vi "Fix File Name.vi"(11 "Config Name":string) -> (3 "File Name":string)   [LabVIEW 2020, in "Negentropic IDE.lvlib"]
uses:
  Negentropic IDE.lvlib
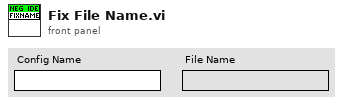
[diagram p1: front panel]
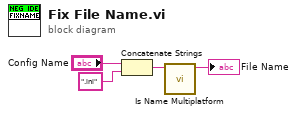
[diagram p0: block diagram]
diagram:
  n1 = Concatenate Strings("Config Name", ".ini" ("string")) -> (w2:string)
  n2 = call <vilib>:"Is Name Multiplatform.vi"("filename"=w2) -> ("suggested filename"=→"File Name":string)  [unwired: 6 in, 4 out]
